vi "TopLevel.vi"() -> ()   [LabVIEW 2020]
uses:
  ProligentResultProcessor/Datawarehouse/GetDestinationFolder.vi
  ProligentResultProcessor/Datawarehouse/SetDestinationFolder.vi
  ProligentResultProcessor/Datawarehouse/SetGenerationTime.vi
  ProligentResultProcessor/Datawarehouse/SetIntegrationMetaData.vi
  ProligentResultProcessor/Datawarehouse/SetBaseFileName.vi
  ProligentResultProcessor/Datawarehouse/SetDataSourceFingerprint.vi
  ProligentResultProcessor/Datawarehouse/GetGenerationTime.vi
  ProligentResultProcessor/Datawarehouse/GetIntegrationMetaData.vi
  ProligentResultProcessor/Datawarehouse/GetBaseFileName.vi
  ProligentResultProcessor/Datawarehouse/GetDataSourceFingerprint.vi
  ProligentResultProcessor/Datawarehouse/GetTopProcessRuns.vi
  ProligentResultProcessor/Datawarehouse/GetProductUnits.vi
  ProligentResultProcessor/ProcessRun/ProcessRun.lvclass
  ProligentResultProcessor/ProductUnit/ProductUnit.lvclass
  ProligentResultProcessor/Datawarehouse/Datawarehouse.lvclass
panel:
  out "Passed":bool
  out "error out":errorcluster
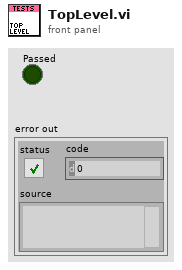
[diagram p1: front panel]
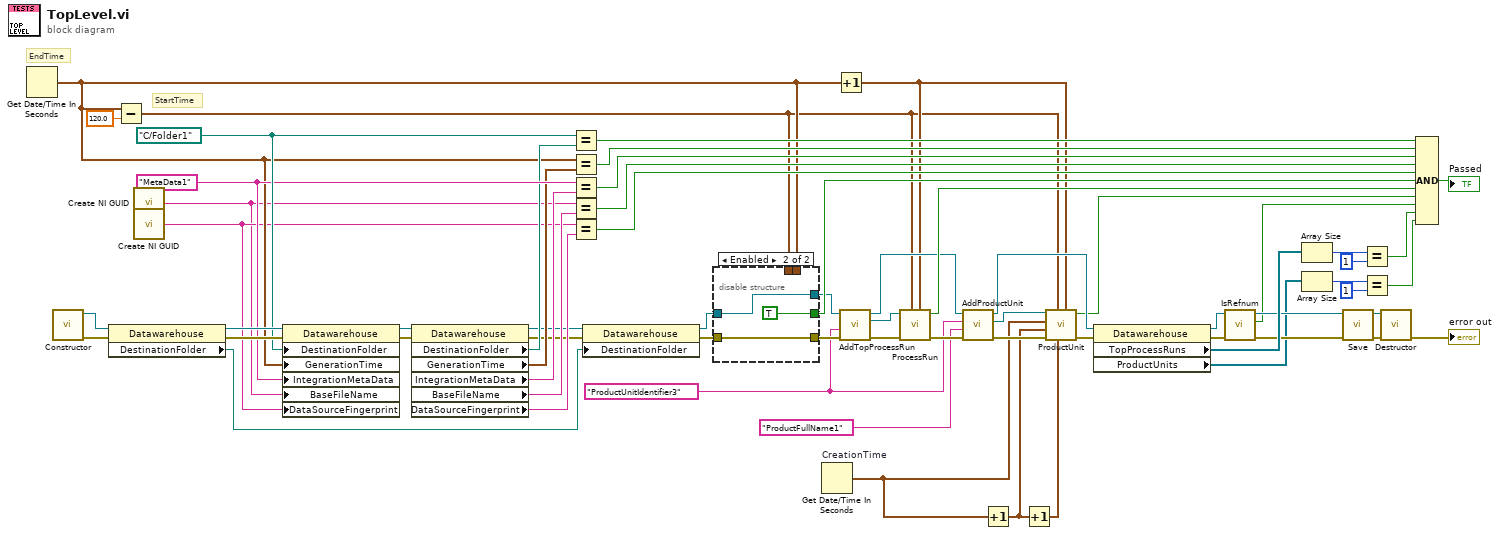
[diagram p0: block diagram]
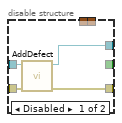
[diagram p2: hidden frame]
diagram:
  w9 = "ProductUnitIdentifier3"
  w56 = "MetaData1"
  w57 = path "C:/Folder1"
  # "EndTime"
  # "StartTime"
  n1 = Get Date/Time In Seconds ("Final Time")() -> (seconds since 1Jan1904=w8:timestamp)
  n2 = call "Constructor.vi"() -> ("error out"=w60:errorcluster, "Datawarehouse"=w61:refnum<class "Datawarehouse.lvclass">)  [unwired: 10 in]
  n3 = property class="Datawarehouse"(reference=w61, error in=w60) -> (reference out=w58:refnum<class "Datawarehouse.lvclass">, error out=w59:errorcluster, "DestinationFolder"=w35:path)
  n4 = Subtract(x=w8, y=120.0) -> (x-y=w7:timestamp)
  n5 = call <vilib>:"Create NI GUID.vi"() -> ("NI GUID"=w1:string)
  n6 = call <vilib>:"Create NI GUID.vi"() -> ("NI GUID"=w3:string)
  n7 = property class="Datawarehouse"(reference=w58, error in=w59, "DestinationFolder"=w57, "GenerationTime"=w8, "IntegrationMetaData"=w56, "BaseFileName"=w1, "DataSourceFingerprint"=w3) -> (reference out=w44:refnum<class "Datawarehouse.lvclass">, error out=w43:errorcluster)
  n8 = property class="Datawarehouse"(reference=w44, error in=w43) -> (reference out=w37:refnum<class "Datawarehouse.lvclass">, error out=w36:errorcluster, "DestinationFolder"=w42:path, "GenerationTime"=w41:timestamp, "IntegrationMetaData"=w40:string, "BaseFileName"=w39:string, "DataSourceFingerprint"=w38:string)
  n9 = Equal?(x=w57, y=w42) -> (x = y?=w55:bool)
  n10 = Equal?(x=w8, y=w41) -> (x = y?=w54:bool)
  n11 = Equal?(x=w56, y=w40) -> (x = y?=w53:bool)
  n12 = Equal?(x=w1, y=w39) -> (x = y?=w51:bool)
  n13 = Equal?(x=w3, y=w38) -> (x = y?=w50:bool)
  n14 = property class="Datawarehouse"(reference=w37, error in=w36, "DestinationFolder"=w35) -> (reference out=w23:refnum<class "Datawarehouse.lvclass">, error out=w26:errorcluster)
  n15 = disable-structure shown="Enabled" {
    disable-tunnel: w26 -> [w68 w69]
    disable-tunnel: [w65 w69] -> w25
    disable-tunnel: w8 -> [_ _]
    disable-tunnel: w7 -> [_ _]
    disable-tunnel: [_ TRUE] -> w24
    disable-tunnel: w23 -> [w67 w71]
    disable-tunnel: [w66 w71] -> w22
    frame Disabled {
      n16 = call "AddDefect.vi"("error in"=w68, "Datawarehouse in"=w67) -> ("error out"=w65:errorcluster, "Datawarehouse out"=w66:refnum<class "Datawarehouse.lvclass">)  [unwired: 7 in, 1 out]
    }
    frame Enabled {
    }
  }
  n17 = Get Date/Time In Seconds "CreationTime"() -> (seconds since 1Jan1904=w6:timestamp)
  n18 = Increment(x=w8) -> (x+1=w12:timestamp)
  n19 = call "AddTopProcessRun.vi"("error in"=w25, "ProductUnitIdentifier"=w9, "Datawarehouse in"=w22) -> ("error out"=w49:errorcluster, "TopProcessRun"=w45:refnum<class "ProcessRun.lvclass">, "Datawarehouse out"=w15:refnum<class "Datawarehouse.lvclass">)  [unwired: 6 in]
  n20 = call "ProcessRun.vi"("EndTime"=w12, "StartTime"=w7, "error in"=w49, "ProcessRun"=w45) -> ("error out"=w17:errorcluster, "Passed"=w34:bool)  [unwired: 6 in]
  n21 = call "AddProductUnit.vi"("error in"=w17, "ProductFullName (Generic_Product)"="ProductFullName1" ("ProductFullName"), "ProductUnitIdentifier"=w9, "Datawarehouse in"=w15) -> ("error out"=w16:errorcluster, "ProductUnit"=w11:refnum<class "ProductUnit.lvclass">, "Datawarehouse out"=w14:refnum<class "Datawarehouse.lvclass">)  [unwired: 5 in]
  n22 = Increment(x=w6) -> (x+1=w5:timestamp)
  n23 = Increment(x=w5) -> (x+1=w4:timestamp)
  n24 = call "ProductUnit.vi"("EndTime"=w12, "ScrappedTime"=w4, "StartTime"=w7, "error in (no error)"=w16, "ManufacturingTime"=w5, "CreationTime"=w6, "ProductUnit in"=w11) -> ("error out"=w13:errorcluster, "Passed"=w2:bool)  [unwired: 3 in]
  n25 = property class="Datawarehouse"(reference=w14, error in=w13) -> (reference out=w30:refnum<class "Datawarehouse.lvclass">, error out=w48:errorcluster, "TopProcessRuns"=w47:refnum<class "ProcessRun.lvclass">[], "ProductUnits"=w18:refnum<class "ProductUnit.lvclass">[])
  n26 = call "IsRefnum.vi"("error in"=w48, "Datawarehouse in"=w30) -> ("error out"=w31:errorcluster, "IsRefnum"=w28:bool, "Datawarehouse out"=w29:refnum<class "Datawarehouse.lvclass">)  [unwired: 7 in]
  n27 = Array Size(array=w47) -> (size(s)=w46:i32)
  n28 = Array Size(array=w18) -> (size(s)=w20:i32)
  n29 = call "Save.vi"("error in"=w31, "Datawarehouse in"=w29) -> ("error out"=w62:errorcluster, "Datawarehouse out"=w63:refnum<class "Datawarehouse.lvclass">)  [unwired: 8 in]
  n30 = Equal?(x=w46, y=1) -> (x = y?=w33:bool)
  n31 = Equal?(x=w20, y=1) -> (x = y?=w19:bool)
  n32 = call "Destructor.vi"("error in"=w62, "Datawarehouse"=w63) -> ("error out"=→"error out":errorcluster)  [unwired: 9 in]
  n33 = Compound Arithmetic op=AND(w55, w54, w53, w51, w50, w24, w34, w2, w28, w33, w19) -> (→"Passed":bool)
